vi "Write Text.vi"(5 "Filename Suffix":string, 6 "Extension (.txt)":string=".txt", 7 "Folder":string="src", 8 "error in (no error)":errorcluster, 9 "Content":string, 10 "VI Path in":path, 11 "Directory Path in":path) -> (0 "error out":errorcluster, 2 "VI Path out":path, 3 "Directory Path out":path)   [LabVIEW 2021, in "NI Measurement Plug-In SDK.lvlib"]
uses:
  NI Measurement Plug-In SDK.lvlib
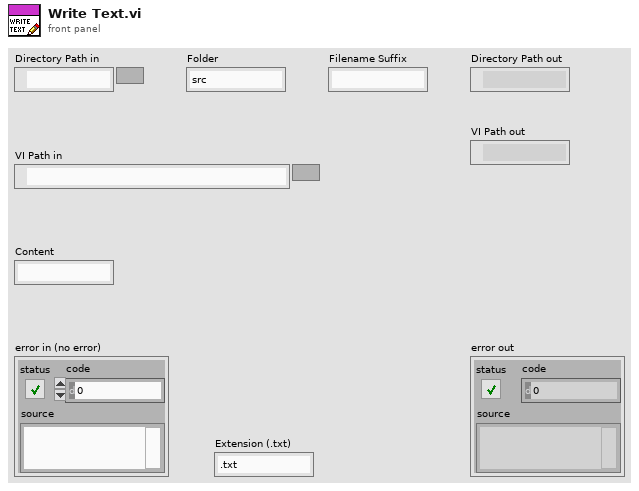
[diagram p1: front panel]
types:
  T1 = enum16{"open", "replace", "create", "open or create", "replace or create", "replace or create with confirmation"}
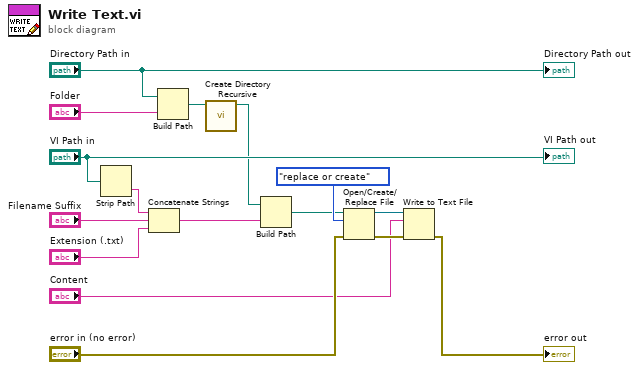
[diagram p0: block diagram]
diagram:
  n1 = Strip Path(path="VI Path in") -> (name=w5:string)  [unwired: 1 out]
  n2 = Concatenate Strings(w5, "Filename Suffix", "Extension (.txt)") -> (w2:string)
  n3 = Build Path(base path="Directory Path in", name or relative path="Folder") -> (appended path=w4:path)
  n4 = call <vilib>:"Create Directory Recursive.vi"("directory"=w4) -> ("directory copy"=w3:path)  [unwired: 4 in, 2 out]
  n5 = Build Path(base path=w3, name or relative path=w2) -> (appended path=w1:path)
  n6 = Open/Create/Replace File(file path (use dialog)=w1, error in="error in (no error)", operation (0:open)=T1."replace or create") -> (refnum out=w12:refnum<file>, error out=w16:errorcluster)  [unwired: 3 in, 1 out]
  n7 = Write to Text File(file (use dialog)=w12, text="Content", error in=w16) -> (error out=→"error out":errorcluster)  [unwired: 1 in, 2 out]
  "Directory Path out" <- "Directory Path in"
  "VI Path out" <- "VI Path in"
